vi "get_sweep_duration.vi"(8 "error in (no error)":errorcluster, 11 "ScanModeMG091111IntrinsicImaging in":refnum<class "ImagingModeMG091111IntrinsicImaging.lvclass">) -> (0 "error out":errorcluster, 2 "sweep duration":dbl[unit], 3 "ScanModeMG091111IntrinsicImaging out":refnum<class "ImagingModeMG091111IntrinsicImaging.lvclass">)   [LabVIEW 2010, in "ImagingModeMG091111IntrinsicImaging.lvclass"]
uses:
  ImagingModeMG091111IntrinsicImaging.lvclass
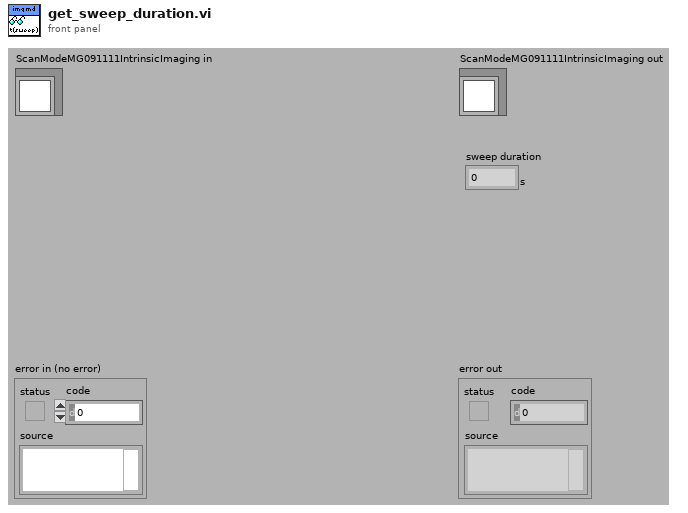
[diagram p1: front panel]
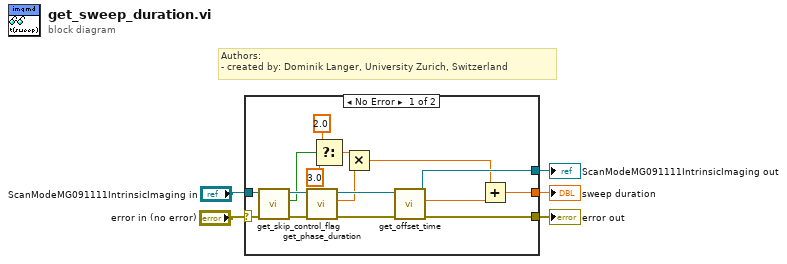
[diagram p0: block diagram]
diagram:
  # "Authors: \n- created by: Dominik Langer, University Zurich, Switzerland"
  n1 = case shown="No Error" "error in (no error)" {
    selector: "error in (no error)" -> [w10 w23]
    tunnel: [w12 w23] -> w4
    tunnel: [w19 w22] -> w2
    tunnel: "ScanModeMG091111IntrinsicImaging in" -> [w8 w22]
    tunnel: [w11 _] -> w1
    frame No Error {
      n2 = call-dynamic "get_skip_control_flag.vi"("error in (no error)"=w10, "ScanModeMG091111IntrinsicImaging in"=w8) -> ("error out"=w9:errorcluster, "skip control?"=w6:bool, "ScanModeMG091111IntrinsicImaging out"=w7:refnum<class "ImagingModeMG091111IntrinsicImaging.lvclass">)  [unwired: 7 in]
      n3 = call-dynamic "get_phase_duration.vi"("error in (no error)"=w9, "ScanModeMG091111IntrinsicImaging in"=w7) -> ("error out"=w21:errorcluster, "phase duration"=w16:dbl[unit], "ScanModeMG091111IntrinsicImaging out"=w20:refnum<class "ImagingModeMG091111IntrinsicImaging.lvclass">)  [unwired: 7 in]
      n4 = Select(t=2.0, s=w6, f=3.0) -> (s? t:f=w15:dbl)
      n5 = Multiply(x=w15, y=w16) -> (x*y=w13:dbl[unit])
      n6 = call-dynamic "get_offset_time.vi"("error in (no error)"=w21, "ScanModeMG091111IntrinsicImaging in"=w20) -> ("error out"=w12:errorcluster, "offset time"=w14:dbl[unit], "ScanModeMG091111IntrinsicImaging out"=w19:refnum<class "ImagingModeMG091111IntrinsicImaging.lvclass">)  [unwired: 7 in]
      n7 = Add(x=w13, y=w14) -> (x+y=w11:dbl[unit])
    }
    frame Error {
    }
  }
  "error out" <- w4
  "ScanModeMG091111IntrinsicImaging out" <- w2
  "sweep duration" <- w1
